vi "Acquire.vi"(8 "error in (no error)":errorcluster, 11 "DAQ Hardware In":T1={"Task"="", "Max"=5.0, "min"=-5.0, "Samples Rate"=1000.0, "Channels"=[]} {"min" format="%0.2f"; "Max" format="%0.2f"}) -> (0 "error out":errorcluster, 2 "Data":waveform(dbl)[](array[waveform]), 3 "DAQ Hardware Out":T1={"Task"="", "Max"=5.0, "min"=-5.0, "Samples Rate"=1000.0, "Channels"=[]} {"min" format="%0.2f"; "Max" format="%0.2f"}, 5 "Data":dbl[][](array[numeric]))   [LabVIEW 2014, in "NIDAQ.lvlib"]
uses:
  NIDAQ.lvlib
  DAQHardware.ctl
  <vilib>/DAQmx/read.llb/DAQmx Read (Analog 1D Wfm NChan NSamp).vi
  <resource>/objmgr/daqmx.rc
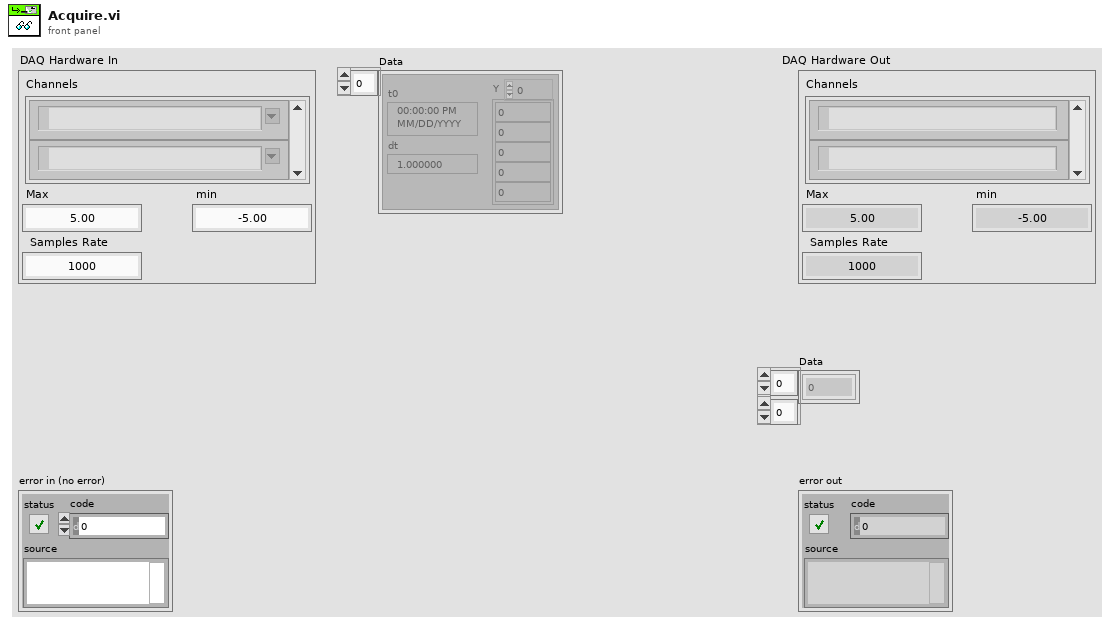
[diagram p1: front panel]
types:
  T1 = typedef "NIDAQ.lvlib/DAQHardware.ctl" = cluster{"Task":refnum<k21>, "Max":dbl, "min":dbl, "Samples Rate":dbl, "Channels":tag[]}
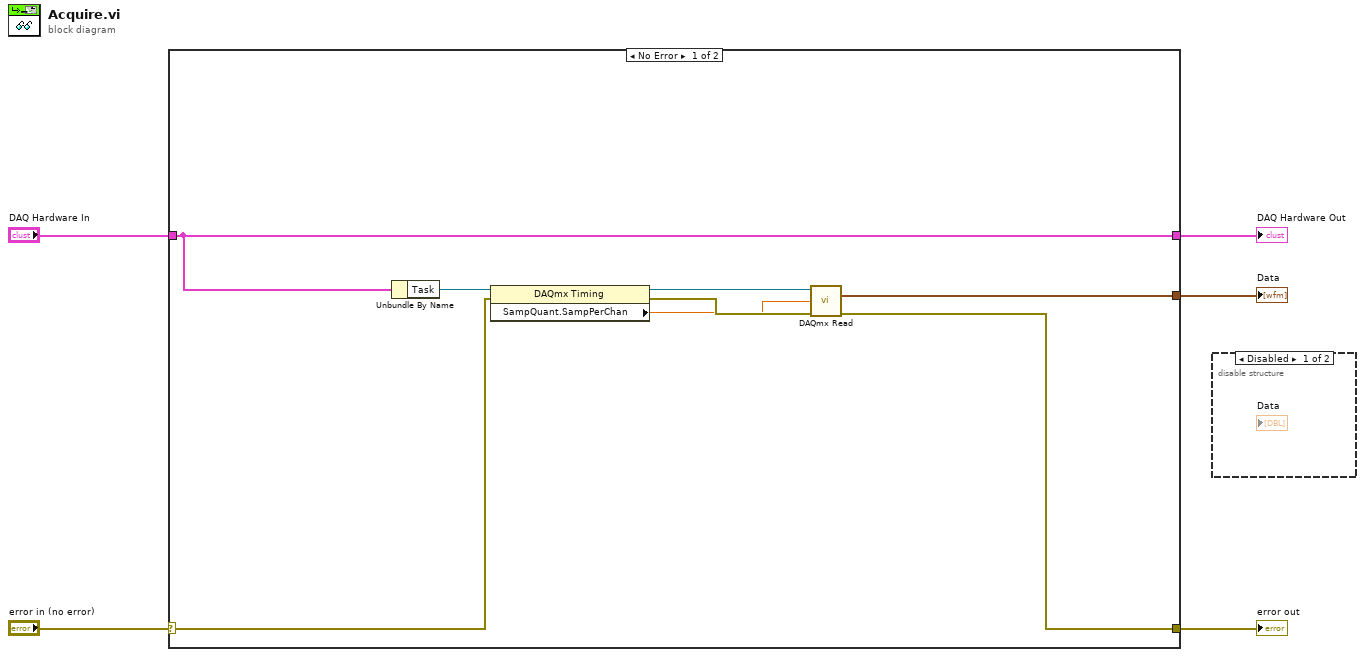
[diagram p0: block diagram]
diagram:
  n1 = case shown="No Error" "error in (no error)" {
    selector: "error in (no error)" -> [w10 w15]
    tunnel: [w8 w15] -> w4
    tunnel: "DAQ Hardware In" -> [w13 w14]
    tunnel: [w13 w14] -> w2
    tunnel: [w7 _] -> w1
    frame No Error {
      n2 = Unbundle By Name(w13) -> ("Task"=w12:refnum<k21>)
      n3 = property class="DAQmx Timing"(reference=w12, error in=w10) -> (reference out=w11:refnum<k21>, error out=w9:errorcluster, "SampQuant.SampPerChan"=w6:dbl)
      n4 = call-poly <vilib>:"DAQmx Read.vi"("task/channels in"=w11, "number of samples per channel"=w6, "error in"=w9) -> ("data"=w7:waveform(dbl)[], "error out"=w8:errorcluster)  [unwired: 10 in, 1 out]
    }
    frame Error {
    }
  }
  "error out" <- w4
  "DAQ Hardware Out" <- w2
  "Data" <- w1
  n5 = disable-structure shown="Disabled" {
    frame Disabled {
    }
    frame Enabled {
    }
  }
